vi "VCS Get Current Must Ex.vi"(8 "error in (no error)":errorcluster, 11 "axis in":cluster{"keyHandle":u32, "nodeId":u16}={"keyHandle"=0, "nodeId"=1}) -> (0 "error out":errorcluster, 2 "currentMust":i32, 3 "axis out":cluster{"keyHandle":u32, "nodeId":u16}={"keyHandle"=0, "nodeId"=1})   [LabVIEW 2017, in "maxonEPOS.lvlib"]
doc: "<B>VCS Get Current Must</B> reads the current mode demand value."
uses:
  Examples/maxonEPOS.lvlib
  SSI_Tool/InstrumentsInterfaces/Motordriver/maxon EPOS/Resources/EposCmd.dll
  SSI_Tool/InstrumentsInterfaces/Motordriver/maxon EPOS/Resources/EposCmd64.dll
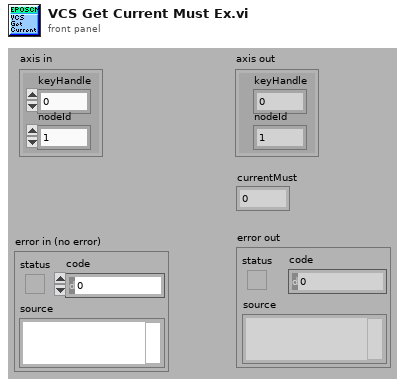
[diagram p1: front panel]
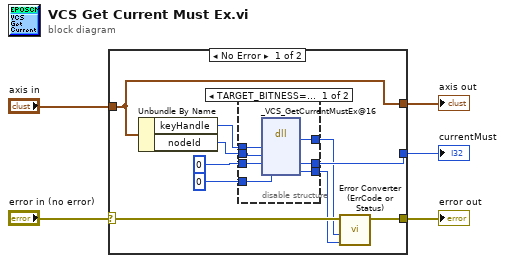
[diagram p0: block diagram]
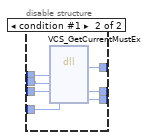
[diagram p2: hidden frame]
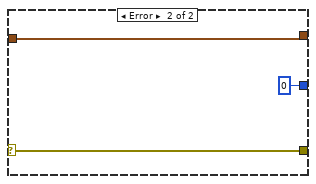
[diagram p3: hidden frame]
diagram:
  n1 = case shown="No Error" "error in (no error)" {
    selector: "error in (no error)" -> [w14 w32]
    tunnel: [w13 w32] -> w4
    tunnel: [w15 i16 0 ("pCurrentMust")] -> w3
    tunnel: "axis in" -> [w7 w31]
    tunnel: [w7 w31] -> w1
    frame No Error {
      n2 = Unbundle By Name(w7) -> ("keyHandle"=w11:u32, "nodeId"=w10:u16)
      n3 = disable-structure shown="TARGET_BITNESS==32, default" {
        disable-tunnel: [w22 w29] -> w15
        disable-tunnel: [w21 w28] -> w12
        disable-tunnel: w11 -> [w20 w27]
        disable-tunnel: w10 -> [w19 w26]
        disable-tunnel: 0 ("pCurrentMust") -> [w18 w25]
        disable-tunnel: u32 0 ("pErrorCode") -> [w17 w24]
        disable-tunnel: [w16 w23] -> w6
        frame condition #0 (active) {
          n4 = dll-call lib="C:/workspace/project/scancon/sw/SSI_Tool/InstrumentsInterfaces/Motordriver/maxon EPOS/Resources/EposCmd.*" fn="_VCS_GetCurrentMustEx@16" ("EposCmd.dll:_VCS_GetCurrentMust@16")("KeyHandle"=w20, "NodeId"=w19, "pCurrentMust"=w18, "pErrorCode"=w17) -> ("Rückgabetyp"=w16:i32, "pCurrentMust"=w22:i32, "pErrorCode"=w21:u32)  [unwired: 5 in, 2 out]
        }
        frame condition #1 {
          n5 = dll-call lib="C:/Sources/LabVIEW/maxon EPOS/Resources/EposCmd64.*" fn="VCS_GetCurrentMustEx" ("EposCmd.dll:_VCS_GetCurrentMust@16")("KeyHandle"=w27, "NodeId"=w26, "pCurrentMust"=w25, "pErrorCode"=w24) -> ("Rückgabetyp"=w23:i32, "pCurrentMust"=w29:i32, "pErrorCode"=w28:u32)  [unwired: 5 in, 2 out]
        }
      }
      n6 = call "Error Converter (ErrCode or Status).vi"("error code"=w12, "return type"=w6, "error in (no error)"=w14) -> ("error out"=w13:errorcluster)  [unwired: 7 in]
    }
    frame Error {
    }
  }
  "currentMust" <- w3
  "error out" <- w4
  "axis out" <- w1
